vi "Read Style.vi"(8 "error in (no error)":errorcluster, 11 "Control in":refnum<class "Control.lvclass">) -> (0 "error out":errorcluster, 1 "Style name":string, 2 "Style index":T1, 3 "Control out":refnum<class "Control.lvclass">)   [LabVIEW 2013, in "Control.lvclass"]
doc: "Accessor VI for the control class"
uses:
  Control.lvclass
  Typedefs/TypeDef_Styles.ctl
  Control.lvclass/Control.ctl
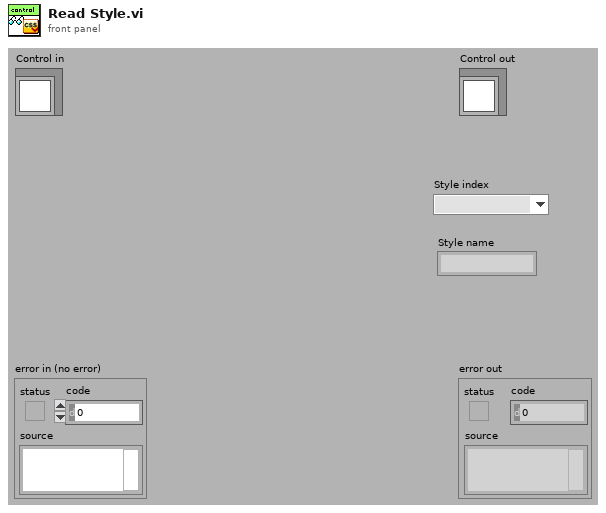
[diagram p1: front panel]
types:
  T1 = typedef "Control.lvclass/TypeDef_Styles.ctl" = u16
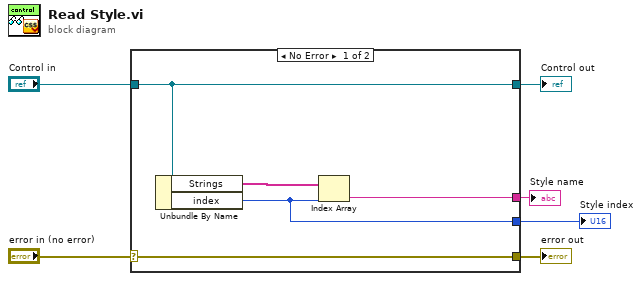
[diagram p0: block diagram]
diagram:
  n1 = case shown="No Error" "error in (no error)" {
    selector: "error in (no error)" -> [w11 w12]
    tunnel: [w11 w12] -> w5
    tunnel: [w10 w13] -> w3
    tunnel: "Control in" -> [w10 w13]
    tunnel: [w7 _] -> w2
    tunnel: [w8 _] -> w1
    frame No Error {
      n2 = Unbundle By Name(w10) -> ("Strings"=w9:string[], "index"=w7:u16)
      n3 = Index Array(array=w9, index=w7) -> (element=w8:string)
    }
    frame Error {
    }
  }
  "error out" <- w5
  "Control out" <- w3
  "Style index" <- w2
  "Style name" <- w1
